vi "Actuator-DM.vi"(0 "Input Cluster":T2={"Manual Mode (T)"=FALSE, "Distance Units"="mm", "Distance"=10, "Power (25)"=50, "Direction (T: Fwd)"=FALSE, "Next Action"=0} {"Next Action" items=["Brake", "Coast"]}, 2 "NXT":T4={"error"={"status"=FALSE, "code"=0, "source"=""}, "address"="", "NXT #"=-1, "Show Error"=TRUE, "Connection"=4} {"Connection" items=["USB", "Bluetooth", "USB then Bluetooth", "Last Connection", "Preference"]}, 3 "Output Port (All Ports)":T3=3 items=["Port A", "Port B", "Port C", "All Ports"]) -> (4 "NXT dup":T4={"error"={"status"=FALSE, "code"=0, "source"=""}, "address"="", "NXT #"=-1, "Show Error"=TRUE, "Connection"=4} {"Connection" items=["USB", "Bluetooth", "USB then Bluetooth", "Last Connection", "Preference"]})   [LabVIEW 2009]
uses:
  <vilib>/NXT/Subs/LVHSConnector.ctl
  <vilib>/NXT/Subs/MotorOutput.ctl
  <vilib>/NXT/Block Support/NXT_Motor.BreakNextAction.ctl
  <vilib>/NXT/Block Support/NXT_ButtonSelector.ctl
  <vilib>/NXT/Dual Mode Library/Sensors/readNXTButton.vi
  <vilib>/NXT/Dual Mode Library/Motors/MotorBrake.vi
  <vilib>/NXT/Dual Mode Library/Motors/MotorCoast.vi
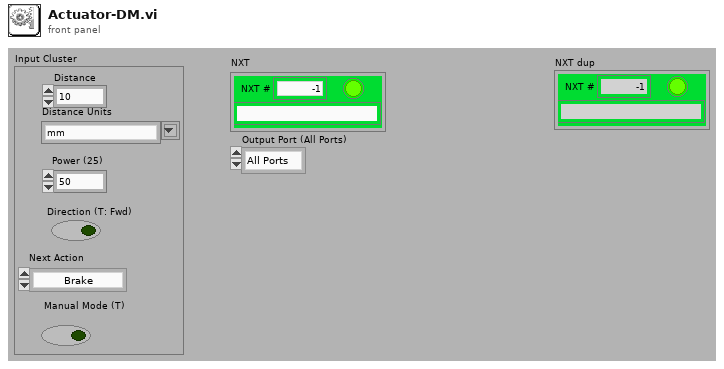
[diagram p1: front panel]
types:
  T1 = typedef "NXT_Motor.BreakNextAction.ctl" = u16
  T2 = cluster{"Manual Mode (T)":bool, "Distance Units":string, "Distance":i32, "Power (25)":i32, "Direction (T: Fwd)":bool, "Next Action":T1}
  T3 = typedef "MotorOutput.ctl" = u8
  T4 = typedef "LVHSConnector.ctl" = cluster{"error":errorcluster, "address":string, "NXT #":i32, "Show Error":bool, "Connection":u16}
  T5 = typedef "NXT_ButtonSelector.ctl" = u16
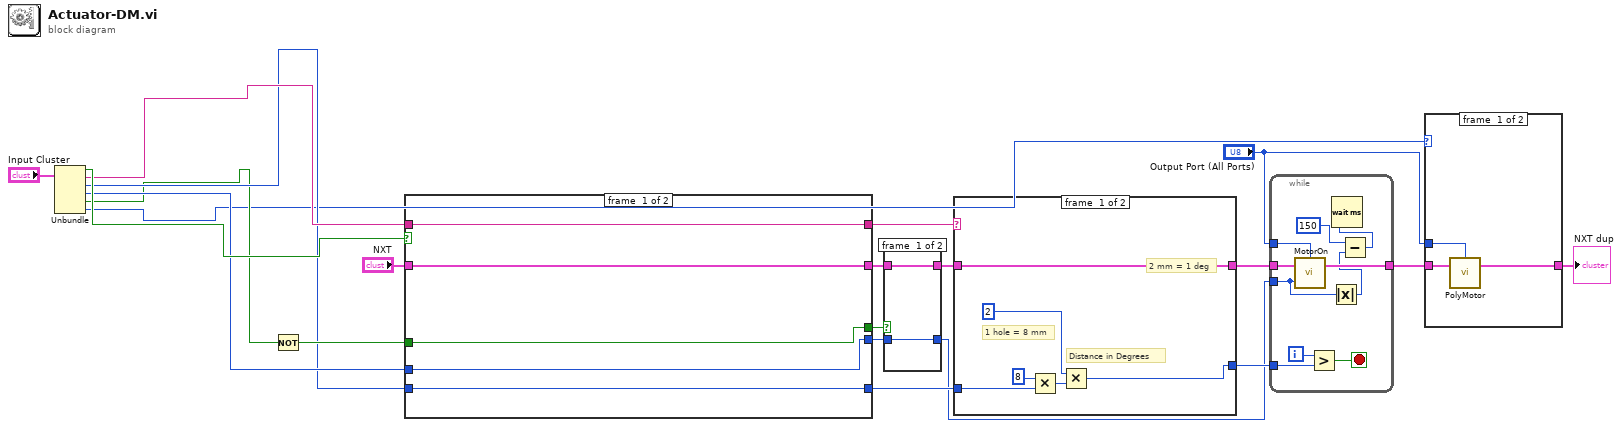
[diagram p0: block diagram]
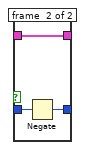
[diagram p2: hidden frame]
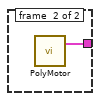
[diagram p3: hidden frame]
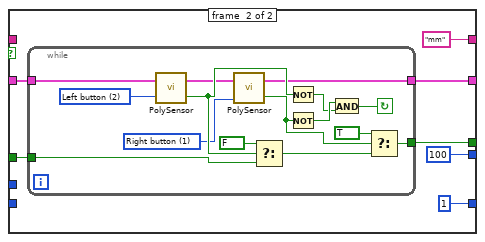
[diagram p4: hidden frame]
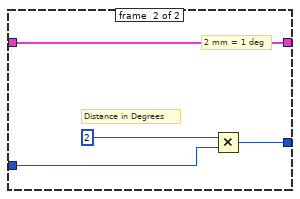
[diagram p5: hidden frame]
diagram:
  n1 = Unbundle("Input Cluster") -> ("Manual Mode (T)"=w6:bool, "Distance Units"=w5:string, "Distance"=w3:i32, "Power (25)"=w4:i32, "Direction (T: Fwd)"=w2:bool, "Next Action"=w1:T1)
  n2 = Not(x=w2) -> (.not. x?=w20:bool)
  n3 = case shown="False" w6 {
    tunnel: w20 -> [w22 w33]
    tunnel: [w26 "mm" ("Distance Units")] -> w21
    tunnel: w5 -> [w26 _]
    tunnel: [w25 1 ("Distance in Millimetres (10)")] -> w10
    tunnel: w3 -> [w25 _]
    tunnel: [w24 100 ("Power (25)")] -> w9
    tunnel: w4 -> [w24 _]
    tunnel: "NXT" -> [w23 w29]
    tunnel: [w23 w28] -> w15
    tunnel: [w22 w27] -> w19
    frame #0 {
    }
    frame #1 {
      n4 = while {
        tunnel: w33 -> [w45]
        tunnel: [w44] -> w27
        tunnel: w29 -> [w35]
        tunnel: [w34] -> w28
        stop <- w39 continue-if-true
        w37 = T5 1 items=["Enter button"=3, "Left button"=2, "Right button"=1] ("Button (Enter button)")
        w38 = T5 2 items=["Enter button"=3, "Left button"=2, "Right button"=1] ("Button (Enter button)")
        n5 = call-poly <vilib>:"PolySensor.vi"("Button (Enter button)"=w38, "NXT"=w35) -> ("Yes/No"=w47:bool, "NXT"=w36:T4)  [unwired: 1 in]
        n6 = call-poly <vilib>:"PolySensor.vi"("Button (Enter button)"=w37, "NXT"=w36) -> ("Yes/No"=w46:bool, "NXT"=w34:T4)  [unwired: 1 in]
        n7 = Select(t=FALSE, s=w47, f=w45) -> (s? t:f=w48:bool)
        n8 = Not(x=w47) -> (.not. x?=w40:bool)
        n9 = Not(x=w46) -> (.not. x?=w41:bool)
        n10 = And(x=w41, y=w40) -> (x .and. y?=w39:bool)
        n11 = Select(t=TRUE, s=w46, f=w48) -> (s? t:f=w44:bool)
      }
    }
  }
  n12 = case shown="False" w19 {
    tunnel: [w50 w53] -> w16
    tunnel: w15 -> [w50 w53]
    tunnel: w9 -> [w49 w52]
    tunnel: [w49 w51] -> w8
    frame #0 {
    }
    frame #1 {
      n13 = Negate(x=w52) -> (-x=w51:i32)
    }
  }
  n14 = case shown="\"mm\", Default" w21 {
    tunnel: [w58 w62] -> w11
    tunnel: w10 -> [w55 w61]
    tunnel: [w54 w60] -> w13
    tunnel: w16 -> [w54 w60]
    frame #0 {
      # "1 hole = 8 mm"
      # "2 mm = 1 deg"
      # "Distance in Degrees"
      n15 = Multiply(x=8, y=w55) -> (x*y=w56:i32)
      n16 = Multiply(x=2, y=w56) -> (x*y=w58:i32)
    }
    frame #1 {
      # "2 mm = 1 deg"
      # "Distance in Degrees"
      n17 = Multiply(x=2, y=w61) -> (x*y=w62:i32)
    }
  }
  n18 = while {
    tunnel: "Output Port (All Ports)" -> [w73]
    tunnel: w13 -> [w72]
    tunnel: [w71] -> w12
    tunnel: w8 -> [w65]
    tunnel: w11 -> [w70]
    i -> [w68]
    stop <- w69 stop-if-true
    n19 = call <vilib>:"MotorOn.vi"("Power (75)"=w65, "NXT"=w72, "Output Port (All Ports)"=w73) -> ("NXT"=w71:T4)  [unwired: 1 in]
    n20 = Greater?(x=w68, y=w70) -> (0:w69:bool)
    n21 = Absolute Value(x=w65) -> (abs(x)=w66:i32)
    n22 = Subtract(x=u8 150, y=w66) -> (x-y=w64:i32)
    n23 = Wait (ms)(milliseconds to wait=w64) -> ()  [unwired: 1 out]
  }
  n24 = case shown="0, Default" w1 {
    tunnel: "Output Port (All Ports)" -> [w76 _]
    tunnel: [w75 w77] -> w18
    tunnel: w12 -> [w74 _]
    frame #0 {
      n25 = call-poly <vilib>:"PolyMotor.vi"("NXT"=w74, "Port (All Ports)"=w76) -> ("NXT"=w75:T4)  [unwired: 2 in]
    }
    frame #1 {
      n26 = call-poly <vilib>:"PolyMotor.vi"() -> ("NXT"=w77:T4)  [unwired: 4 in]
    }
  }
  "NXT dup" <- w18
